vi "Get cRIO-9063 Modules Info.vi"(8 "error in":errorcluster) -> (0 "error out":errorcluster, 2 "cRIO Modules":T1[](array[typedef]) {"Serial Number" format="%.0x"; "Vendor and Module ID" format="%.0x"})   [LabVIEW 2015]
doc: "This VI retrieves the current configuration of modules in a cRIO-9072 chassis including the module type and serial number of each module. It uses a subVI to store a list of available modules and their model ID codes. This subVI can be updated to support new C series modules being released.\n\nThe VI downloads a bitstream to the FPGA in order to query the modules. This bitstream replaces any bitstream (FPGA VI) currently running on the FPGA."
uses:
  Controls/cRIO Module Info.ctl
  <vilib>/FPGAPlugInAG/Dynamic/niLvFpga_Close_Dynamic.vi
  <vilib>/FPGAPlugInAG/Dynamic/niLvFpga_Run_Dynamic.vi
  <vilib>/rvi/interface/nirviCloseFPGA/nirviCloseFPGA.xnode
  <vilib>/rvi/interface/nirviMethod/nirviMethod.xnode
  Module Detection.lvclass
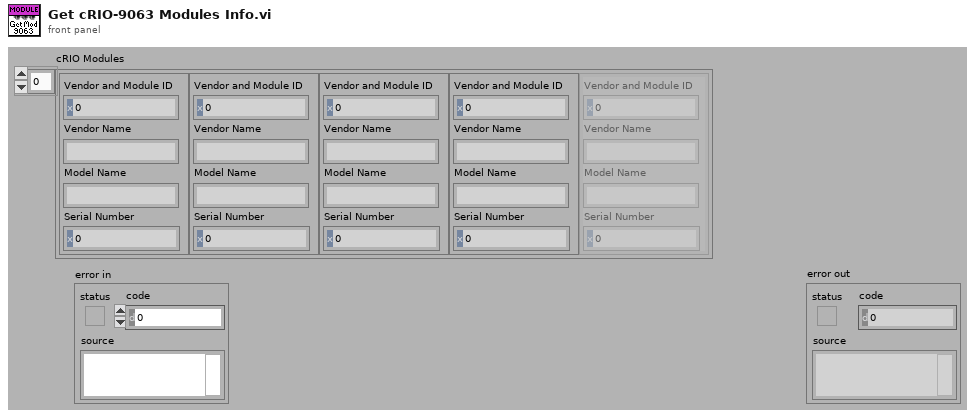
[diagram p1: front panel]
types:
  T1 = typedef "RT Management.lvlib/Module Detection.lvclass/cRIO Module Info.ctl" = cluster{"Vendor and Module ID":u32, "Vendor Name":string, "Model Name":string, "Serial Number":u32}
  T2 = cluster{"Vendor and Module ID":u32, "Vendor Name":string, "Model Name":string, "Serial Number":u32}
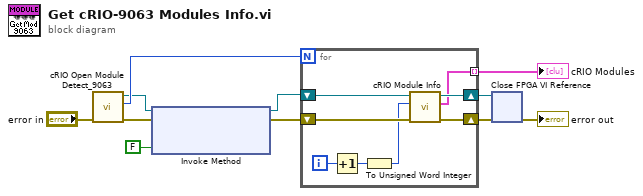
[diagram p0: block diagram]
diagram:
  n1 = call "cRIO Open Module Detect_9063.vi"("error in"="error in") -> ("error out"=w7:errorcluster, "slots"=w8:i32, "Refnum out"=w6:refnum<k20>)  [unwired: 8 in]
  n2 = xnode "Invoke Method"("FPGA VI Reference In"=w6, "error in"=w7, "Wait Until Done (F)"=FALSE) -> ("FPGA VI Reference Out"=w10:refnum<k20>, "error out"=w9:errorcluster)
  n3 = for {
    N: w8 -> [_]
    shift-right: [w16] -> w1
    shift-left: w10 -> [w19]
    shift-right: [w17] -> w3
    shift-left: w9 -> [w18]
    tunnel: [w12] -> w4 mode=indexing
    i -> [w15]
    n4 = Increment(x=w15) -> (x+1=w14:i32)
    n5 = To Unsigned Word Integer(number=w14) -> (unsigned 16bit integer=w13:u16)
    n6 = call "cRIO Module Info.vi"("error in"=w18, "Module"=w13, "Refnum in"=w19) -> ("error out"=w17:errorcluster, "cRIO Module Info"=w12:T2, "Refnum out"=w16:refnum<k20>)  [unwired: 6 in]
  }
  "cRIO Modules" <- w4
  n7 = xnode "Close FPGA VI Reference"("FPGA VI Reference In"=w1, "error in"=w3) -> ("error out"=→"error out":errorcluster)
